vi "test_MonoMove.vi"(8 "error in":errorcluster, 11 "Monochromator in":refnum<class "Monochromator.lvclass">) -> (0 "error out":errorcluster, 3 "Monochromator out":refnum<class "Monochromator.lvclass">)   [LabVIEW 2020, in "horiba.test.lvlib"]
uses:
  horiba.test.lvlib
  Classes/Mono/Monochromator.lvclass
  <vilib>/addons/_JKI Toolkits/Caraya/classes/Assert/Assert Almost Equal_Float.vi
panel:
  # "Connector Pane"
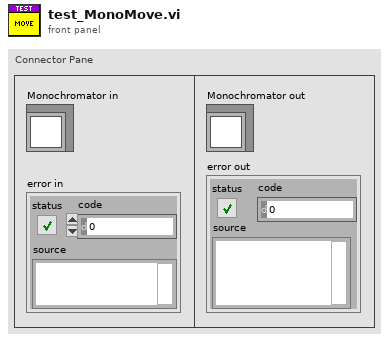
[diagram p1: front panel]
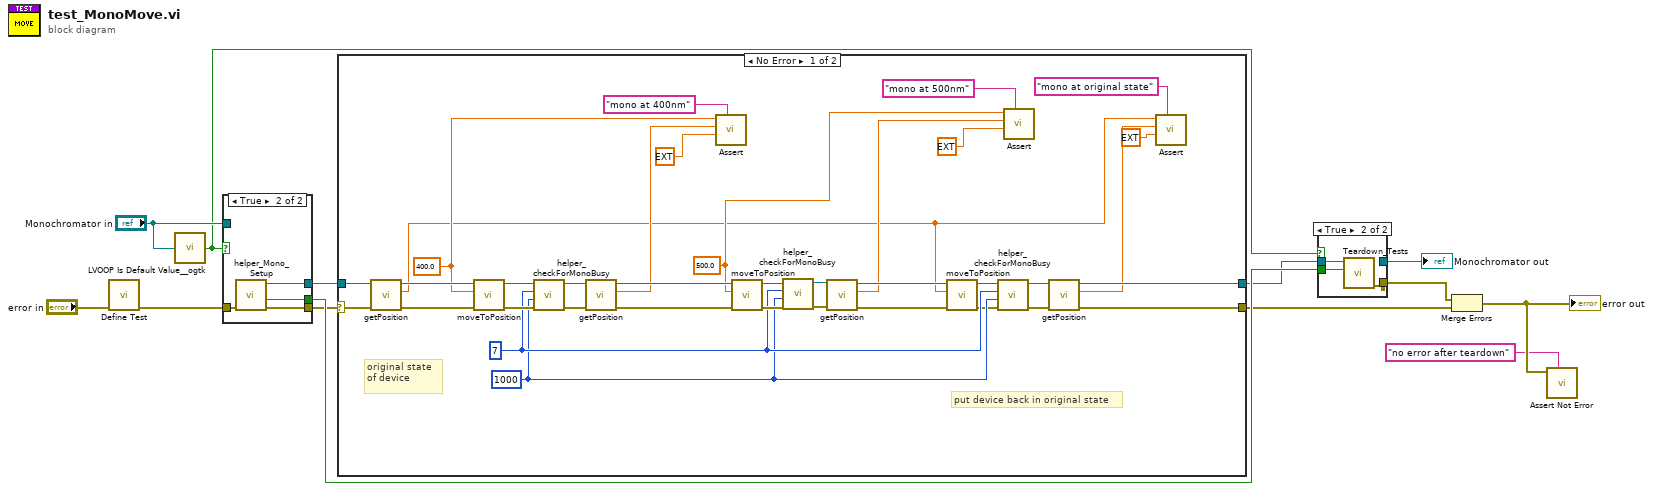
[diagram p0: block diagram]
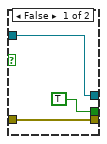
[diagram p2: hidden frame]
diagram:
  n1 = call <vilib>:"Define Test.vi"("error in (no error)"="error in") -> ("error out"=w7:errorcluster)  [unwired: 9 in, 1 out]
  n2 = call <userlib>:"LVOOP Is Default Value__ogtk.vi"("Object"="Monochromator in") -> ("Is Default Value?"=w8:bool)
  n3 = case shown="True" w8 {
    tunnel: w7 -> [w15 w20]
    tunnel: [w15 w19] -> w2
    tunnel: [w16 w18] -> w5
    tunnel: [TRUE ("Module Was Already Running?") w17] -> w10
    tunnel: "Monochromator in" -> [w16 _]
    frame False {
    }
    frame True {
      n4 = call "helper_Mono_Setup.vi"("error in"=w20) -> ("error out"=w19:errorcluster, "Module Was Already Running?"=w17:bool, "Monochromator out"=w18:refnum<class "Monochromator.lvclass">)  [unwired: 7 in, 1 out]
    }
  }
  n5 = case shown="No Error" w2 {
    selector: w2 -> [w49 w58]
    tunnel: [w41 w57] -> w4
    tunnel: w5 -> [w48 w57]
    tunnel: [w40 w58] -> w1
    frame No Error {
      w25 = u32 1000 ("milliseconds to wait")
      w26 = 7
      w43 = 500.0 ("position")
      w47 = 400.0 ("position")
      # "put device back in original state"
      # "original state of device"
      n6 = call "getPosition.vi"("error in (no error)"=w49, "Monochromator in"=w48) -> ("error out"=w54:errorcluster, "wavelength"=w38:dbl, "Monochromator out"=w55:refnum<class "Monochromator.lvclass">)  [unwired: 7 in]
      n7 = call "moveToPosition.vi"("error in (no error)"=w54, "wavelength"=w47, "Monochromator in"=w55) -> ("error out"=w36:errorcluster, "Monochromator out"=w37:refnum<class "Monochromator.lvclass">)  [unwired: 5 in, 2 out]
      n8 = call "helper_checkForMonoBusy.vi"("error in (no error)"=w36, "milliseconds to wait"=w25, "Numeric"=w26, "Monochromator in"=w37) -> ("error out"=w34:errorcluster, "Monochromator out"=w35:refnum<class "Monochromator.lvclass">)  [unwired: 5 in, 1 out]
      n9 = call "getPosition.vi"("error in (no error)"=w34, "Monochromator in"=w35) -> ("error out"=w52:errorcluster, "wavelength"=w46:dbl, "Monochromator out"=w53:refnum<class "Monochromator.lvclass">)  [unwired: 7 in]
      n10 = call-poly <vilib>:"Assert.vi"("Label"="mono at 400nm", "Tolerance"=ext 1.0, "Y"=w46, "X"=w47) -> ()  [unwired: 6 in, 2 out]
      n11 = call "moveToPosition.vi"("error in (no error)"=w52, "wavelength"=w43, "Monochromator in"=w53) -> ("error out"=w33:errorcluster, "Monochromator out"=w32:refnum<class "Monochromator.lvclass">)  [unwired: 5 in, 2 out]
      n12 = call "helper_checkForMonoBusy.vi"("error in (no error)"=w33, "milliseconds to wait"=w25, "Numeric"=w26, "Monochromator in"=w32) -> ("error out"=w31:errorcluster, "Monochromator out"=w30:refnum<class "Monochromator.lvclass">)  [unwired: 5 in, 1 out]
      n13 = call "getPosition.vi"("error in (no error)"=w31, "Monochromator in"=w30) -> ("error out"=w50:errorcluster, "wavelength"=w44:dbl, "Monochromator out"=w51:refnum<class "Monochromator.lvclass">)  [unwired: 7 in]
      n14 = call "moveToPosition.vi"("error in (no error)"=w50, "wavelength"=w38, "Monochromator in"=w51) -> ("error out"=w24:errorcluster, "Monochromator out"=w27:refnum<class "Monochromator.lvclass">)  [unwired: 5 in, 2 out]
      n15 = call "helper_checkForMonoBusy.vi"("error in (no error)"=w24, "milliseconds to wait"=w25, "Numeric"=w26, "Monochromator in"=w27) -> ("error out"=w29:errorcluster, "Monochromator out"=w28:refnum<class "Monochromator.lvclass">)  [unwired: 5 in, 1 out]
      n16 = call-poly <vilib>:"Assert.vi"("Label"="mono at 500nm", "Tolerance"=ext 1.0, "Y"=w44, "X"=w43) -> ()  [unwired: 6 in, 2 out]
      n17 = call "getPosition.vi"("error in (no error)"=w29, "Monochromator in"=w28) -> ("error out"=w40:errorcluster, "wavelength"=w39:dbl, "Monochromator out"=w41:refnum<class "Monochromator.lvclass">)  [unwired: 7 in]
      n18 = call-poly <vilib>:"Assert.vi"("Label"="mono at original state", "Tolerance"=ext 1.0, "Y"=w39, "X"=w38) -> ()  [unwired: 6 in, 2 out]
    }
    frame Error {
    }
  }
  n19 = case shown="True" w8 {
    tunnel: w4 -> [w59 w62]
    tunnel: [_ w61] -> w6
    tunnel: w10 -> [_ w60]
    tunnel: [w59 _] -> w3
    frame False {
    }
    frame True {
      n20 = call "Teardown_Tests.vi"("Module Was Already Running?"=w60, "horiba.lvlib:GenericDevice"=w62) -> ("error out"=w61:errorcluster)  [unwired: 8 in, 1 out]
    }
  }
  "Monochromator out" <- w3
  n21 = Merge Errors(w6, w1) -> (w12:errorcluster)
  "error out" <- w12
  n22 = call <vilib>:"Assert Not Error.vi"("Label"="no error after teardown", "Not Error?"=w12) -> ()  [unwired: 8 in, 2 out]
